vi "Loopback Simulation.vi"() -> ()   [LabVIEW 2013]
uses:
  <vilib>/rvi/DesktopExecutionNode/Execution/niFpgaDEN_Execute.vi
  <vilib>/rvi/DesktopExecutionNode/DesktopExecutionNode.xnode
  <vilib>/NI/I2S-TDM IP/I2S-TDM.lvlib
panel:
  in  "Transmit Samples":u32[](array[numeric])=[0, 0, 0, 0, 0, 0, 0, 0]
  out "Received Samples":u32[](array[numeric])
  out "Receive Buffer":u32(slide) scale=0.0..8.0
  out "Transmit Buffer":u32(slide) scale=0.0..8.0
  in  "Loop Wait":u32(slide)=45 min=10 max=70 step=1 scale=10.0..70.0
  in  "pause":bool
  out "Digital Waveform Graph":digitalwaveform(graph)
  in  "stop":bool
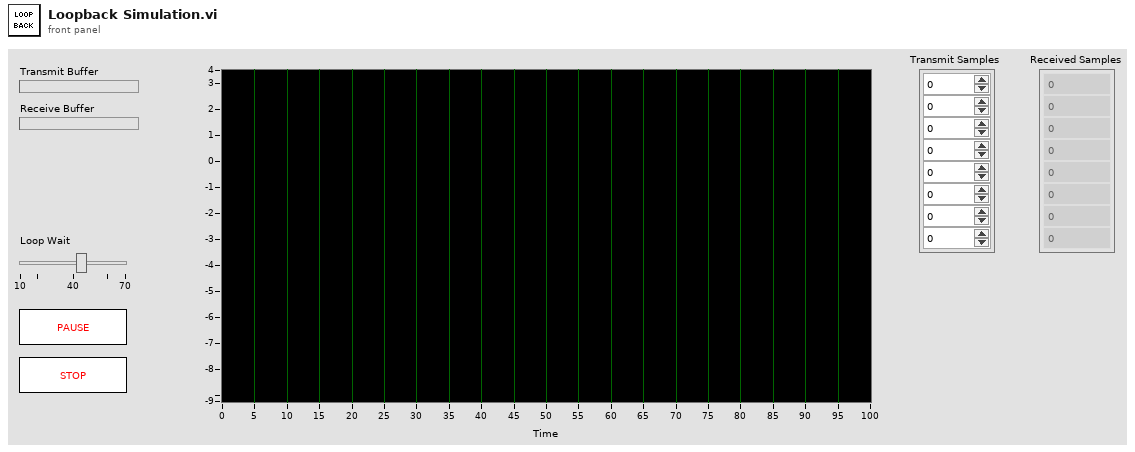
[diagram p1: front panel]
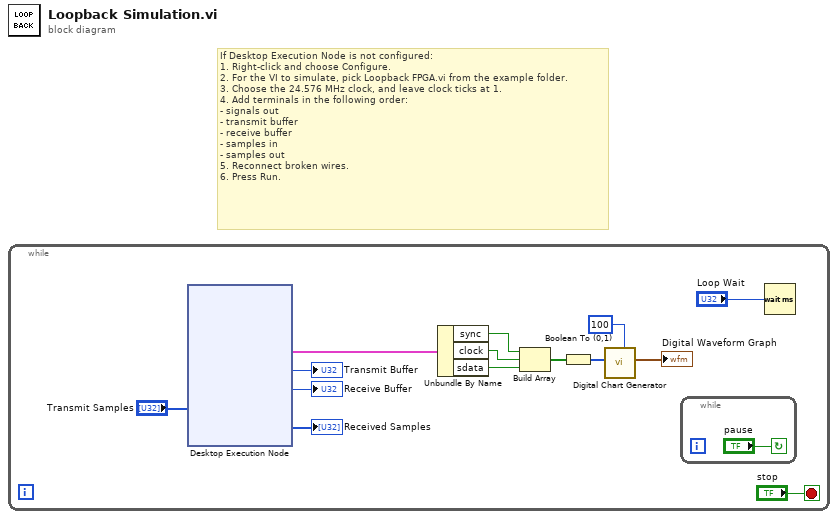
[diagram p0: block diagram]
diagram:
  # "If Desktop Execution Node is not configured:\n1. Right-click and choose Configure.\n2. For the VI to simulate, pick Loopback FPGA.vi from the example folder.\n3. Choose the 24.576 MHz clock, and leave clock ticks at 1.\n4. Add terminals in the following order:\n- signals out\n- transmit buffer\n- receive buffer\n- samples in\n- samples out\n5. Reconnect broken wires.\n6. Press Run."
  n1 = while {
    stop <- "stop" stop-if-true
    n2 = xnode "Desktop Execution Node"("samples in"="Transmit Samples") -> ("signals out"=w2:cluster{"clock":bool, "sync":bool, "sdata":bool}, "transmit buffer"=→"Transmit Buffer":u32, "receive buffer"=→"Receive Buffer":u32, "samples out"=→"Received Samples":u32[])  [unwired: 1 in, 1 out]
    n3 = Unbundle By Name(w2) -> ("sync"=w8:bool, "clock"=w9:bool, "sdata"=w10:bool)
    n4 = Build Array(w8, w9, w10) -> (w12:bool[])
    n5 = Boolean To (0,1)(Boolean=w12) -> (0, 1=w11:i16[])
    n6 = call <vilib>:"Digital Chart Generator.vi"("History Size"=100, "Input"=w11) -> ("Digital Data"=→"Digital Waveform Graph":digitalwaveform)  [unwired: 9 in]
    n7 = while {
      stop <- "pause" continue-if-true
    }
    n8 = Wait (ms)(milliseconds to wait="Loop Wait") -> ()  [unwired: 1 out]
  }
